vi "RP - BUILD MAC CONF FILE.vi"(8 "error in":errorcluster, 9 "RP2 MAC":string, 10 "RP1 MAC":string, 11 "Path":path) -> (0 "error out":errorcluster)   [LabVIEW 2021]
uses:
  <vilib>/Utility/config.llb/Write Key (String).vi
  <vilib>/Utility/config.llb/NI_LVConfig.lvlib
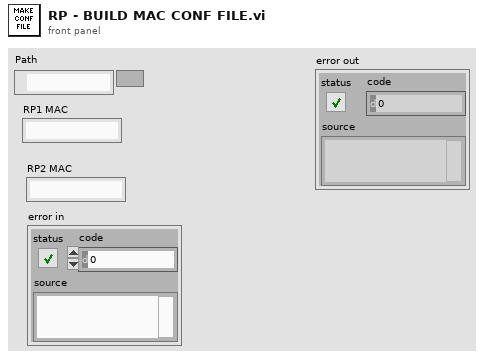
[diagram p1: front panel]
types:
  T1 = typedef "NI_LVConfig.lvlib/Config Data RefNum.ctl" = refnum<k1>
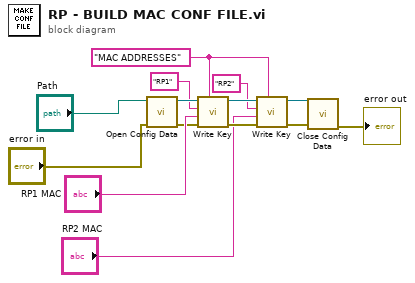
[diagram p0: block diagram]
diagram:
  w7 = "MAC ADDRESSES" ("section")
  n1 = call <vilib>:"Open Config Data.vi"("error in (no error)"="error in", "configuration file path"="Path") -> ("error out"=w10:errorcluster, "refnum"=w13:T1)  [unwired: 7 in, 1 out]
  n2 = call-poly <vilib>:"Write Key.vi"("section"=w7, "error in (no error)"=w10, "value"="RP1 MAC", "key"="RP1", "refnum"=w13) -> ("error out"=w5:errorcluster, "refnum out"=w8:T1)  [unwired: 4 in, 1 out]
  n3 = call-poly <vilib>:"Write Key.vi"("section"=w7, "error in (no error)"=w5, "value"="RP2 MAC", "key"="RP2", "refnum"=w8) -> ("error out"=w2:errorcluster, "refnum out"=w3:T1)  [unwired: 4 in, 1 out]
  n4 = call <vilib>:"Close Config Data.vi"("error in (no error)"=w2, "refnum"=w3) -> ("error out"=→"error out":errorcluster)  [unwired: 8 in, 1 out]
